vi "Write ECAT VARs.vi"(7 "R/W Case":T7, 8 "error in (no error)":errorcluster, 9 "Input FIFO buffer in":dbl[](array[numeric]), 10 "I/O Output Data in":T1 {"BD Refs"."Data Reference" format="%.0x"}, 11 "I/O Imput Vars in":T4[](array[typedef]) {"VS ref" format="%.0x"}) -> (0 "error out":errorcluster, 1 "Input FIFO buffer out":dbl[](array[numeric]), 2 "I/O Output Data out":T1 {"BD Refs"."Data Reference" format="%.0x"}, 3 "I/O Imput Vars out":T4[](array[typedef]) {"VS ref" format="%.0x"})   [LabVIEW 2019, in "SEECD Engine.lvlib"]
uses:
  SEECD Engine.lvlib
  Type Defs/RW Case.ctl
  Type Defs/Generic ECAT Slave IOV Cluster.ctl
  <vilib>/NI VeriStand/Custom Device API/Custom Device Item Ref.ctl
  Shared/Type Defs/UDV Data Type.ctl
  Type Defs/Output Data.ctl
  <vilib>/NI VeriStand/Custom Device API/Block Data Reference.ctl
  <vilib>/NI VeriStand/Custom Device API/Data Reference.ctl
  <vilib>/NI VeriStand/Custom Device API/Global Data Refs.vi
  <vilib>/NI VeriStand/Custom Device API/Custom Device API.lvlib
  Shared/SEECD Shared.lvlib
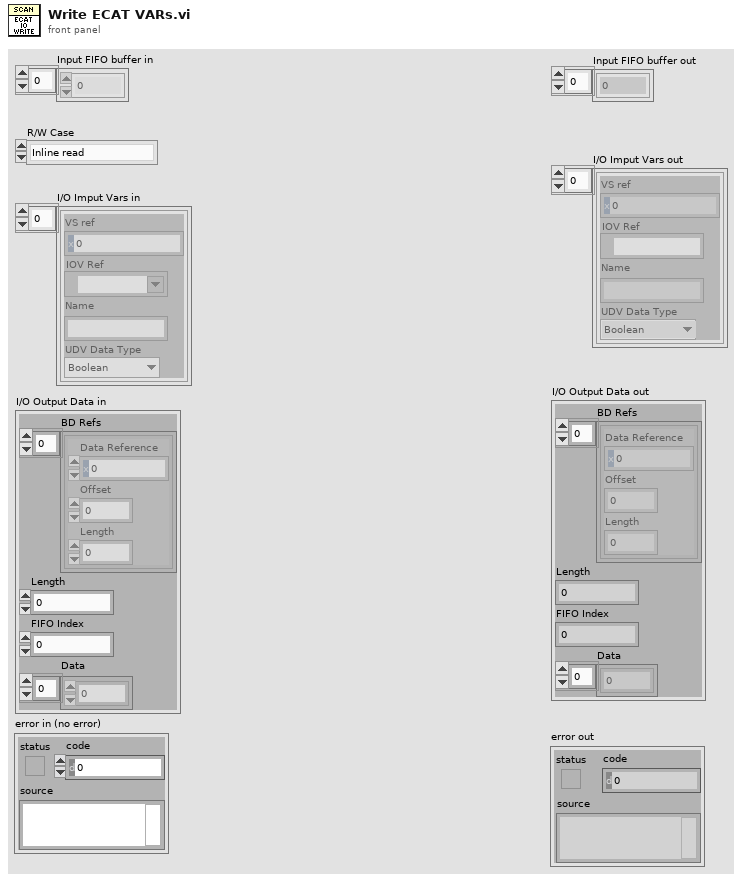
[diagram p1: front panel]
types:
  T1 = typedef "SEECD Engine.lvlib/Output Data.ctl" = cluster{"BD Refs":T2[], "Length":i32, "FIFO Index":i32, "Data":dbl[]}
  T2 = typedef "Custom Device API.lvlib/Block Data Reference.ctl" = cluster{"Data Reference":T3, "Offset":u64, "Length":u64}
  T3 = typedef "Custom Device API.lvlib/Data Reference.ctl" = i32
  T4 = typedef "SEECD Engine.lvlib/Generic ECAT Slave IOV Cluster.ctl" = cluster{"VS ref":T5, "IOV Ref":refnum<k21>, "Name":string, "UDV Data Type":T6}
  T5 = typedef "Custom Device API.lvlib/Custom Device Item Ref.ctl" = u64
  T6 = typedef "SEECD Shared.lvlib/UDV Data Type.ctl" = enum16{"Boolean", "Fixed Point", "Int8", "Int16", "Int32", "Int64", "U32 Bit Field", "UInt8", "UInt16", "UInt32", "UInt64", "Other", "DBL", "SGL"}
  T7 = typedef "SEECD Engine.lvlib/RW Case.ctl" = enum16{"Inline read", "Inline write", "Async - Inline loop read", "Async - Inline loop write", "Async loop (read/write)"}
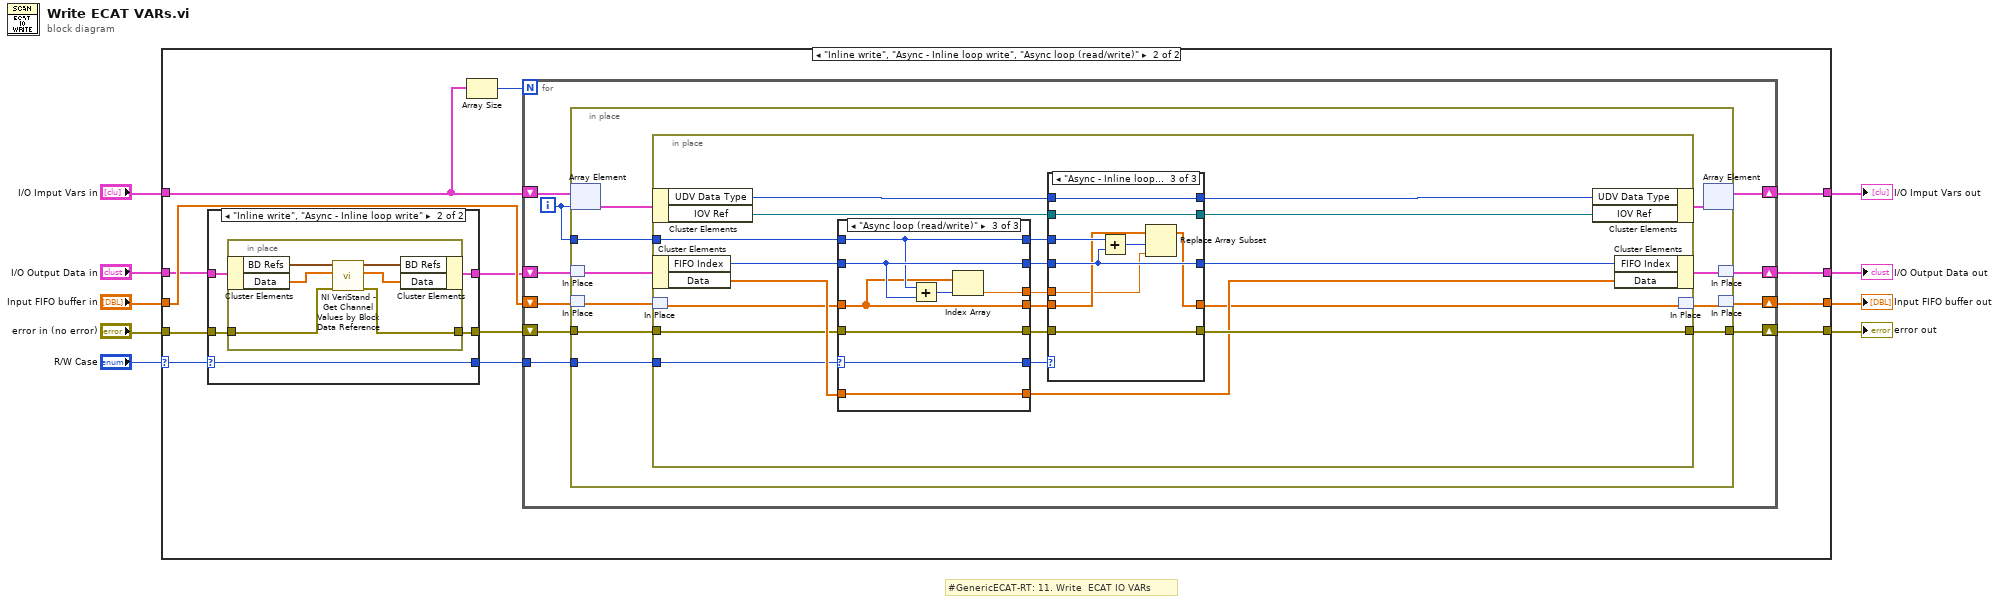
[diagram p0: block diagram]
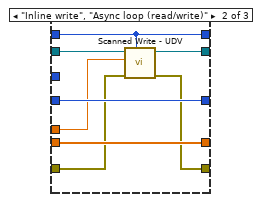
[diagram p4: hidden frame]
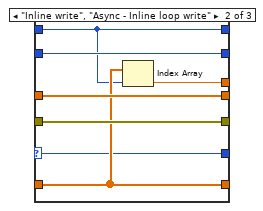
[diagram p6: hidden frame]
diagram:
  # "#GenericECAT-RT: 11. Write  ECAT IO VARs"
  n1 = case shown="\"Inline write\", \"Async - Inline loop write\", \"Async loop (read/write)\"" "R/W Case" {
    selector: "R/W Case" -> [_ w21]
    tunnel: [w11 w26] -> w9
    tunnel: "Input FIFO buffer in" -> [w11 w25]
    tunnel: [w12 w15] -> w2
    tunnel: [w13 w24] -> w3
    tunnel: "I/O Output Data in" -> [w12 w19]
    tunnel: "I/O Imput Vars in" -> [w13 w23]
    tunnel: [w10 w14] -> w7
    tunnel: "error in (no error)" -> [w10 w20]
    frame Default {
    }
    frame "Inline write", "Async - Inline loop write", "Async loop (read/write)" {
      n2 = case shown="\"Inline write\", \"Async - Inline loop write\"" w21 {
        selector: w21 -> [w110 w113]
        tunnel: w19 -> [w111 w117]
        tunnel: w20 -> [w112 w116]
        tunnel: [w112 w115] -> w17
        tunnel: [w111 w114] -> w18
        tunnel: [w110 w113] -> w16
        frame Default {
        }
        frame "Inline write", "Async - Inline loop write" {
          n3 = in-place {
            in-place-border: w116 -> [w119]
            in-place-border: [w118] -> w115
            n4 = in-place-cluster #1(w117) -> ("BD Refs"=w123:T2[], "Data"=w121:dbl[])
            n5 = call <vilib>:"NI VeriStand - Get Channel Values by Block Data Reference.vi"("error in (no error)"=w119, "Values Array in"=w121, "Block Data Ref"=w123) -> ("error out"=w118:errorcluster, "Values Array out"=w120:dbl[], "Block Data Ref dup"=w122:T2[])  [unwired: 6 in]
            n6 = in-place-cluster #1("BD Refs"=w122, "Data"=w120) -> (w114:T1)
          }
        }
      }
      n7 = Array Size(array=w23) -> (size(s)=w22:i32)
      n8 = for {
        N: w22 -> [_]
        shift-right: [w35] -> w24
        shift-left: w23 -> [w36]
        shift-right: [w27] -> w15
        shift-left: w18 -> [w30]
        shift-right: [w33] -> w26
        shift-left: w25 -> [w34]
        shift-right: [w31] -> w14
        shift-left: w17 -> [w32]
        tunnel: w16 -> [w29]
        i -> [w28]
        n9 = in-place {
          in-place-border: w32 -> [w44]
          in-place-border: [w38] -> w31
          in-place-border: w29 -> [w43]
          in-place-border: w28 -> [w42]
          n10 = in-place-array #2(w36, w28) -> (w37:T4)
          n11 = in-place-match #3(w30) -> (w46:T1)
          n12 = in-place-match #4(w34) -> (w45:dbl[])
          n13 = in-place {
            in-place-border: w44 -> [w62]
            in-place-border: w43 -> [w48]
            in-place-border: w42 -> [w63]
            in-place-border: [w59] -> w38
            n14 = in-place-cluster #5(w37) -> ("UDV Data Type"=w64:T6, "IOV Ref"=w54:refnum<k21>)
            n15 = in-place-cluster #6(w46) -> ("FIFO Index"=w66:i32, "Data"=w65:dbl[])
            n16 = in-place-match #7(w45) -> (w50:dbl[])
            n17 = case shown="\"Async loop (read/write)\"" w48 {
              selector: w48 -> [w91 w96 w105]
              tunnel: w63 -> [w89 w97 w106]
              tunnel: w66 -> [w94 w99 w107]
              tunnel: w50 -> [w92 w100 w104]
              tunnel: w62 -> [w90 w101 w109]
              tunnel: w65 -> [w93 w98 w108]
              tunnel: [w94 w99 w107] -> w56
              tunnel: [w93 w98 w108] -> w51
              tunnel: [w90 w101 w109] -> w57
              tunnel: [w92 w100 w104] -> w47
              tunnel: [w91 w96 w105] -> w53
              tunnel: [_ w95 w103] -> w55
              tunnel: [w89 w97 w106] -> w52
              frame Default {
              }
              frame "Inline write", "Async - Inline loop write" {
                n18 = Index Array(array=w98, index=w97) -> (element=w95:dbl)
              }
              frame "Async loop (read/write)" {
                n19 = Add(x=w106, y=w107) -> (x+y=w102:i32)
                n20 = Index Array(array=w104, index=w102) -> (element=w103:dbl)
              }
            }
            n21 = case shown="\"Async - Inline loop write\"" w53 {
              tunnel: w64 -> [w67 w75 w88]
              tunnel: w54 -> [w68 w77 w83]
              tunnel: w56 -> [w69 w78 w85]
              tunnel: w47 -> [w70 w79 w84]
              tunnel: [w70 w79 w82] -> w49
              tunnel: w52 -> [_ _ w86]
              tunnel: [w69 w78 w85] -> w58
              tunnel: [w68 w76 w83] -> w60
              tunnel: [w67 w75 w88] -> w61
              tunnel: w57 -> [w71 w74 w87]
              tunnel: [w71 w73 w87] -> w59
              tunnel: w55 -> [_ w72 w81]
              frame Default {
              }
              frame "Inline write", "Async loop (read/write)" {
                n22 = call "Scanned Write - UDV.vi"("UDV Data Type"=w75, "error in (no error)"=w74, "data in"=w72, "IOV ref in"=w77) -> ("error out"=w73:errorcluster, "IOV ref out"=w76:refnum<k21>)  [unwired: 6 in]
              }
              frame "Async - Inline loop write" {
                n23 = Add(x=w86, y=w85) -> (x+y=w80:i32)
                n24 = Replace Array Subset(array=w84, new element=w81, index=w80) -> (w82:dbl[])
              }
            }
            n25 = in-place-cluster #5("UDV Data Type"=w61, "IOV Ref"=w60) -> (w41:T4)
            n26 = in-place-cluster #6("FIFO Index"=w58, "Data"=w51) -> (w40:T1)
            n27 = in-place-match #7(w49) -> (w39:dbl[])
          }
          n28 = in-place-array #2(w41) -> (w35:T4[])  [unwired: 1 out]
          n29 = in-place-match #3(w40) -> (w27:T1)
          n30 = in-place-match #4(w39) -> (w33:dbl[])
        }
      }
    }
  }
  "Input FIFO buffer out" <- w9
  "error out" <- w7
  "I/O Imput Vars out" <- w3
  "I/O Output Data out" <- w2
